vi "RIB Req - CJB Eathered Error - Normal Operation.vi"(0 "Limits File Path":path, 5 "Results File Path":path, 11 "error in":errorcluster) -> (4 "Results Data Array":string[][](array[string]), 15 "error out":errorcluster)   [LabVIEW 2024]
doc: "Template test"
uses:
  <vilib>/addons/_JKI Toolkits/State Machine/_JKI_lib_State_Machine.llb/Select State(s)_err__jki_lib_state_machine.vi
  <vilib>/addons/_JKI Toolkits/State Machine/_JKI_lib_State_Machine.llb/Select State(s)_bool__jki_lib_state_machine.vi
  <vilib>/addons/_JKI Toolkits/State Machine/_JKI_lib_State_Machine.llb/Periodic Trigger__ogtk__JKI-SM__jki_lib_state_machine.vi
  <userlib>/_OpenG.lib/file/file.llb/Strip Path Extension - String__ogtk.vi
  <vilib>/Utility/file.llb/Read Delimited Spreadsheet (string).vi
  <vilib>/Utility/file.llb/Write Delimited Spreadsheet (string).vi
  <userlib>/_OpenG.lib/file/file.llb/openg_file.lvlib
  <userlib>/_OpenG.lib/appcontrol/appcontrol.llb/openg_application_control.lvlib
  <userlib>/_OpenG.lib/time/time.llb/openg_time.lvlib
panel:
  out "State Value":string
  out "Wait for Start":bool
  out "Normal Operation":bool
  out "Timeout - Start State":dbl(slide) scale=0.0..15.0
  in  "eSTOP 1 State Error Test":string
  in  "eSTOP 1 State Test":string
  in  "Read Start":string
  in  "Read Set":string
  out "Timeout":dbl(slide) scale=0.0..60.0
  in  "eSTOP 1 Error Test":string
  in  "eSTOP 1 Test":string
  in  "connection ID":refnum<k16>
  in  "handle out":u64
  in  "Exit":bool
  # "Normal Operation"
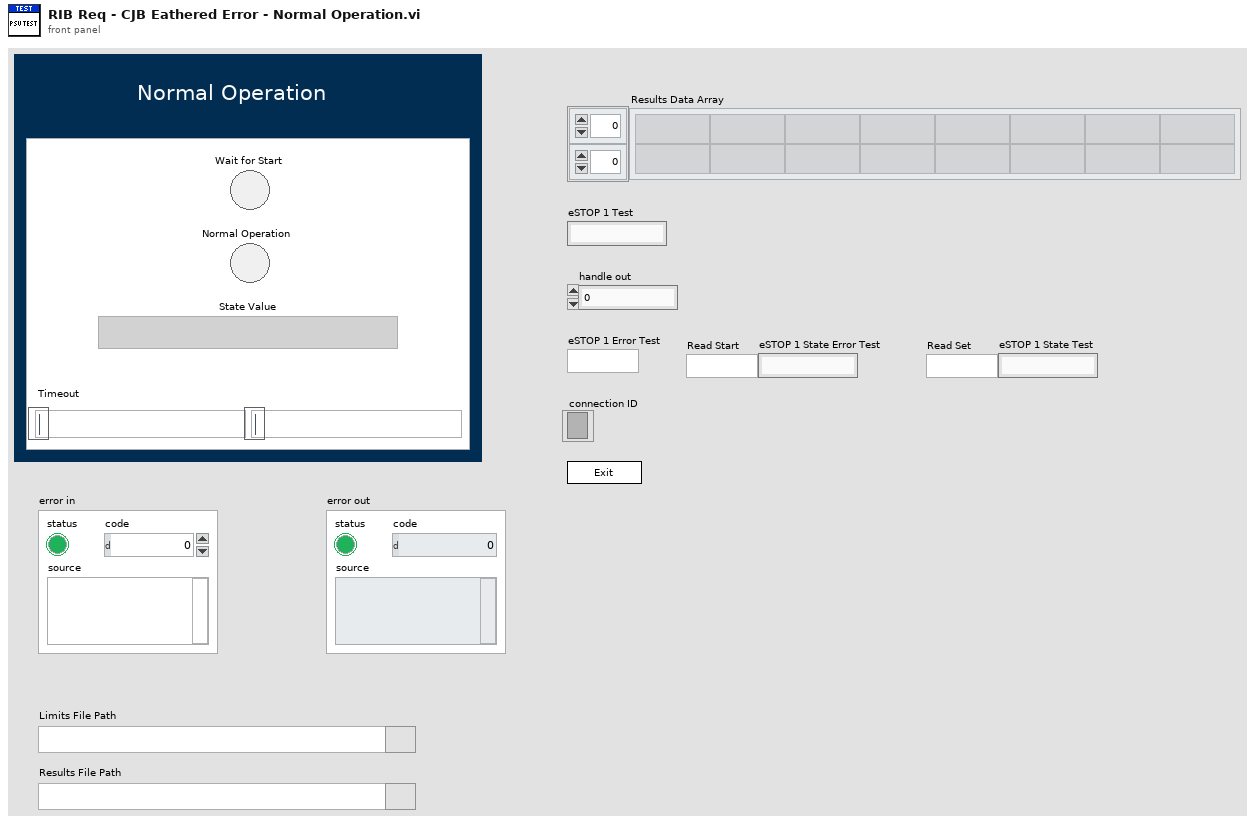
[diagram p1: front panel]
types:
  T1 = enum32{"Invalid", "Standard", "Closed", "Hidden", "Minimized", "Maximized"}
  T2 = enum32{"invalid app kind", "Development System", "Run Time System", "Student Edition", "Embedded LabVIEW", "Evaluation", "Custom"}
  T3 = typedef "FGV - Enum" = enum16{"Cleanup", "Get Data", "Simulator", "Open UDP", "Initialise DAQ", "Initialise I2C"}
  T4 = enum16{"Start Timer", "Get Time", "Pause", "Unpause"}
  T5 = cluster{"Core":cluster{"Current VI Reference":refnum<vi>, "Close Panel on Exit?":bool}, "Limits File Path":path, "Test Limits":string[][], "Results Data Array":string[][], "Results File Path":path, "Voltage":dbl, "connection ID":refnum<k16>, "handle out":u64, "eSTOP 1 Test":string, "eSTOP 1 Error Test":string, "Read Set":string, "Read Start ":string, "eSTOP 1 State Test":string, "eSTOP 1 State Error Test":string, "State Value":string}
  T6 = cluster{"Current VI Reference":refnum<vi>, "Close Panel on Exit?":bool}
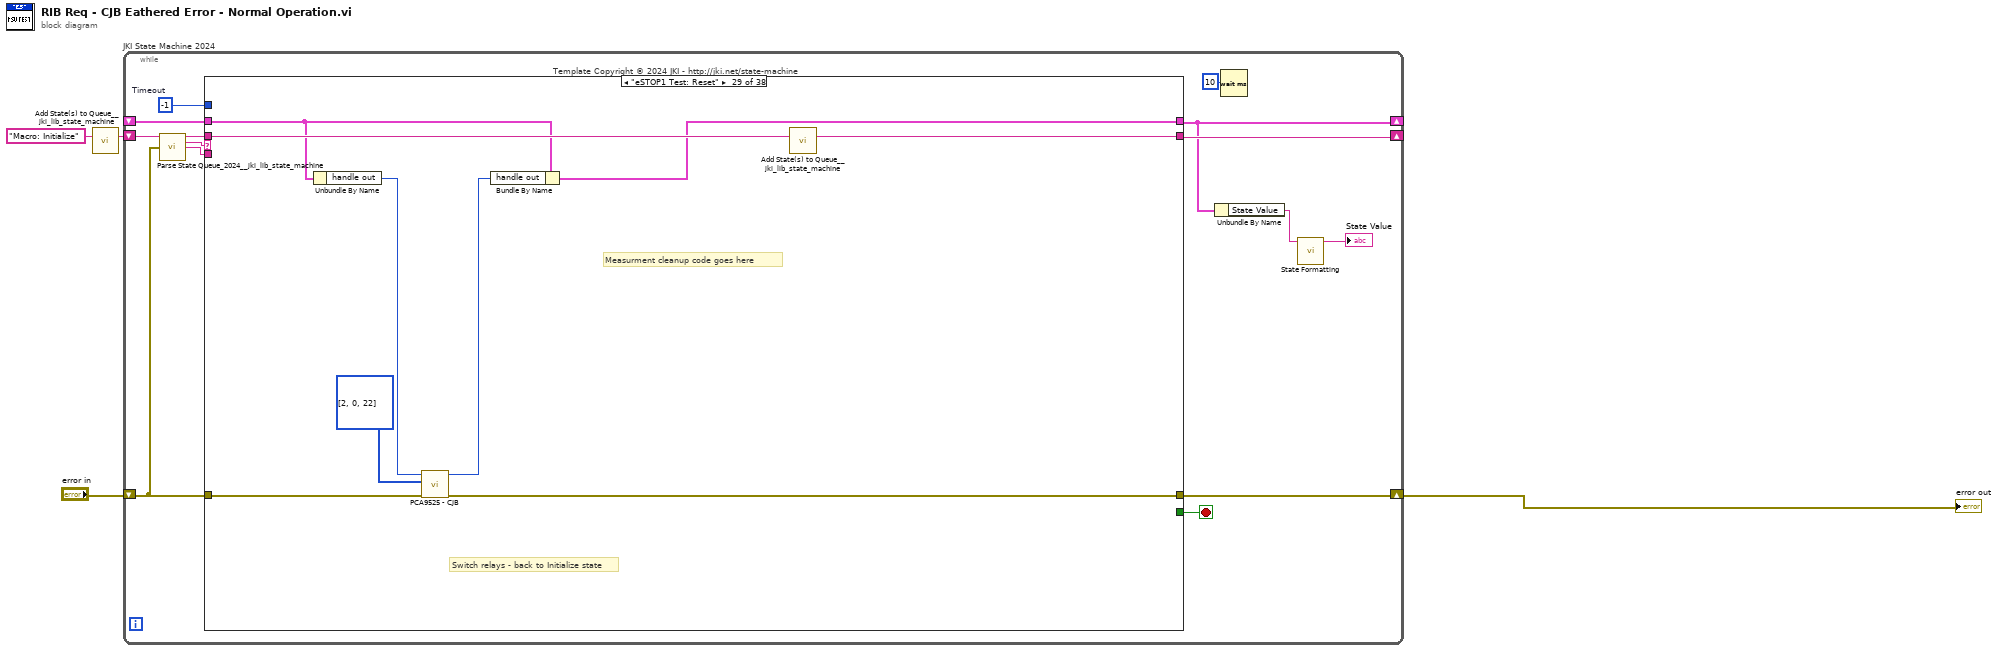
[diagram p0: block diagram]
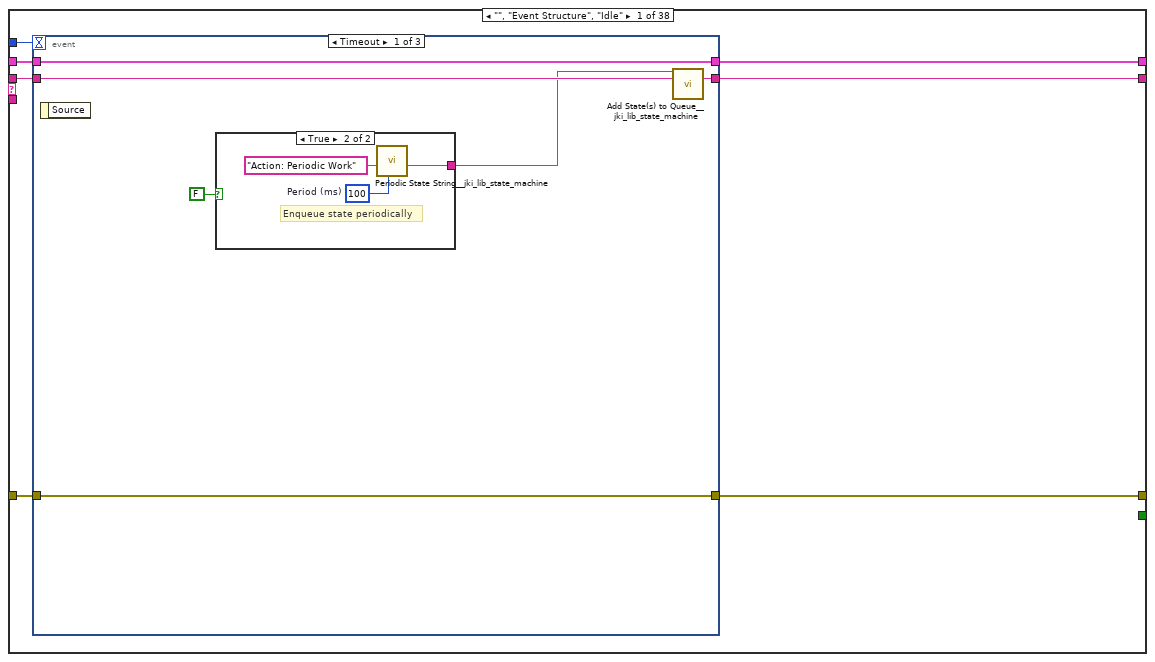
[diagram p2: hidden frame]
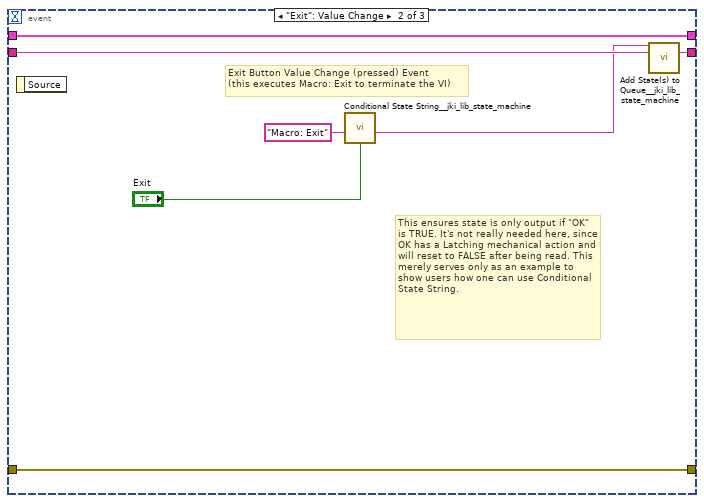
[diagram p4: hidden frame]
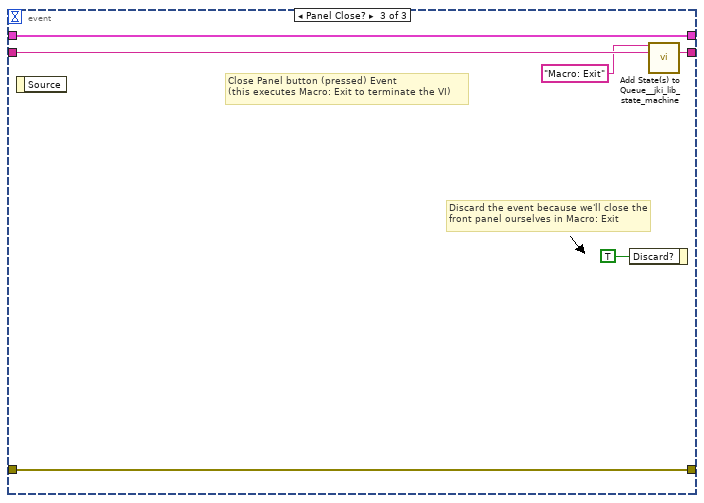
[diagram p5: hidden frame]
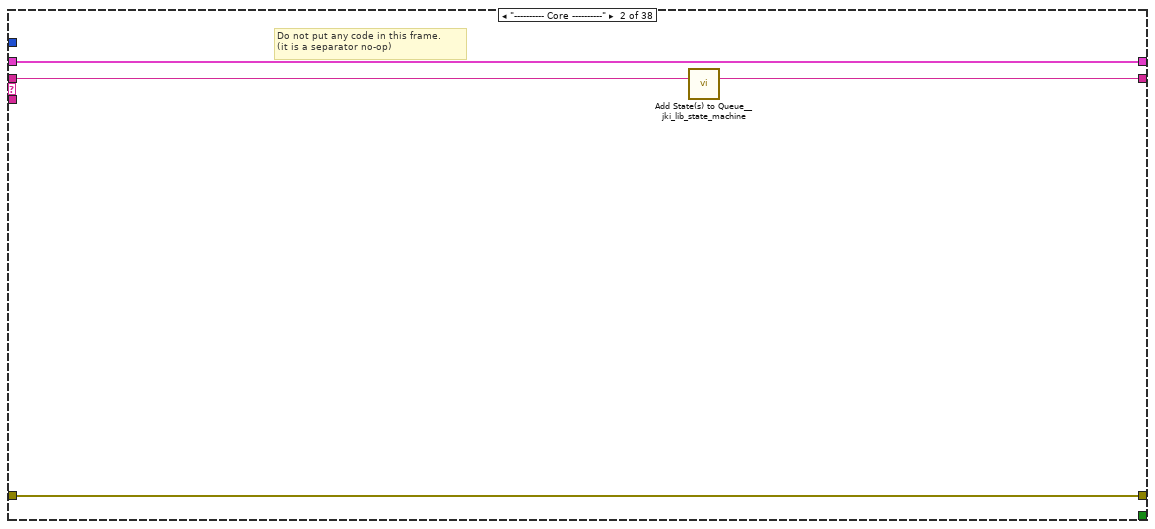
[diagram p6: hidden frame]
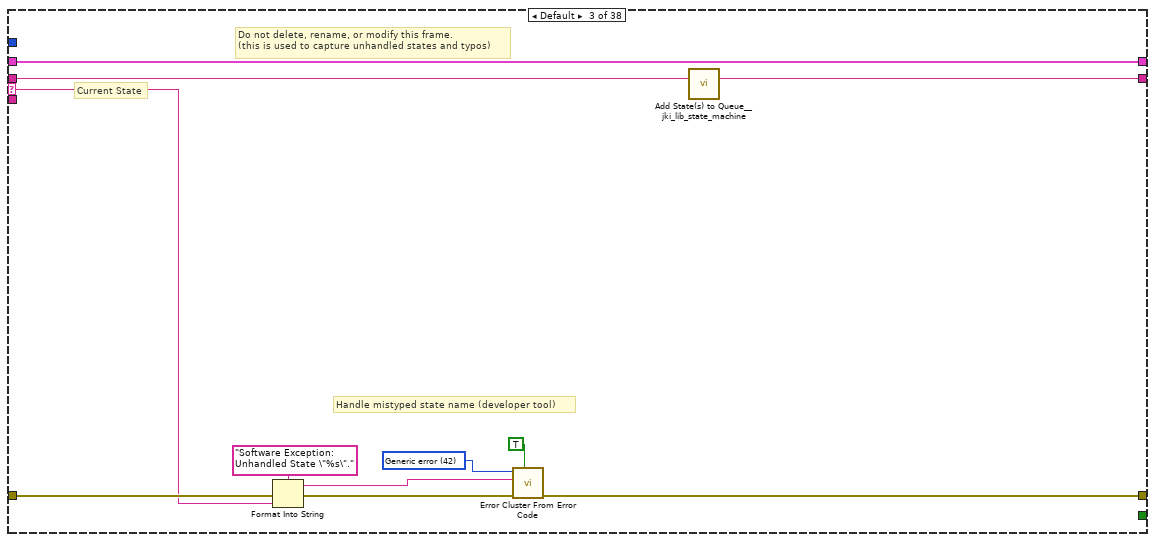
[diagram p7: hidden frame]
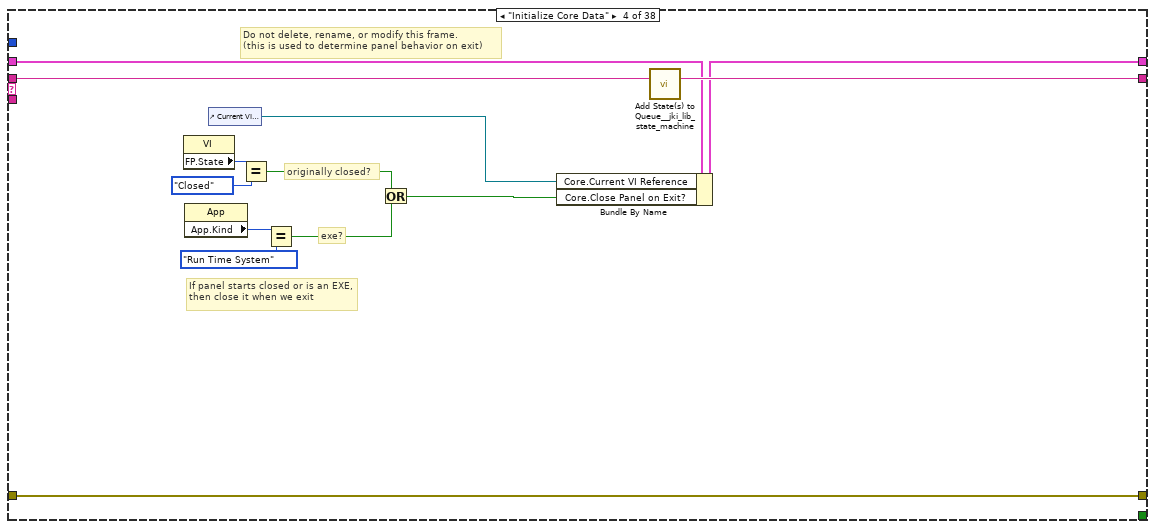
[diagram p8: hidden frame]
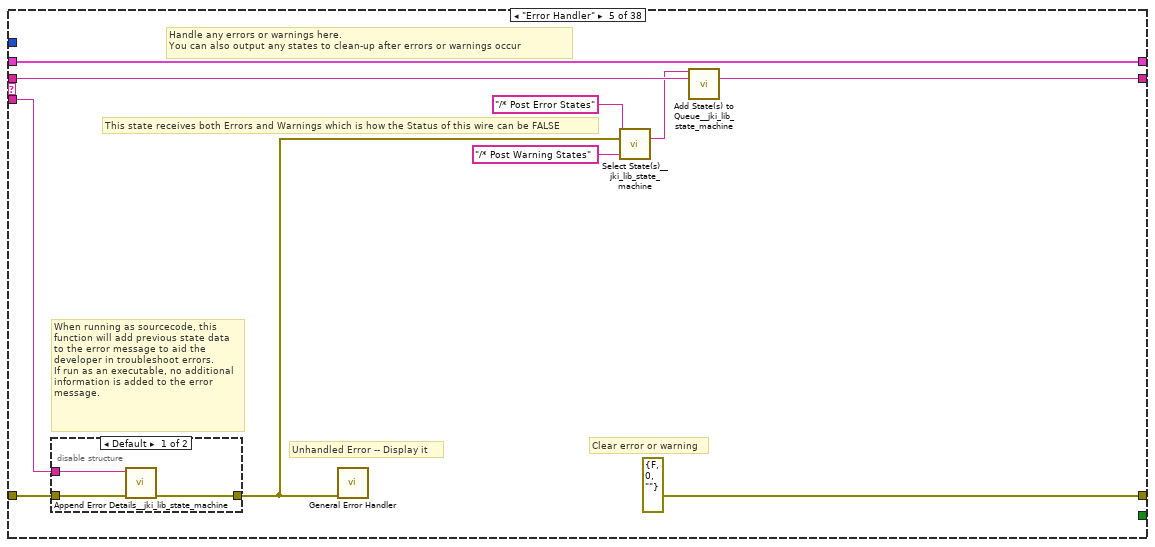
[diagram p9: hidden frame]
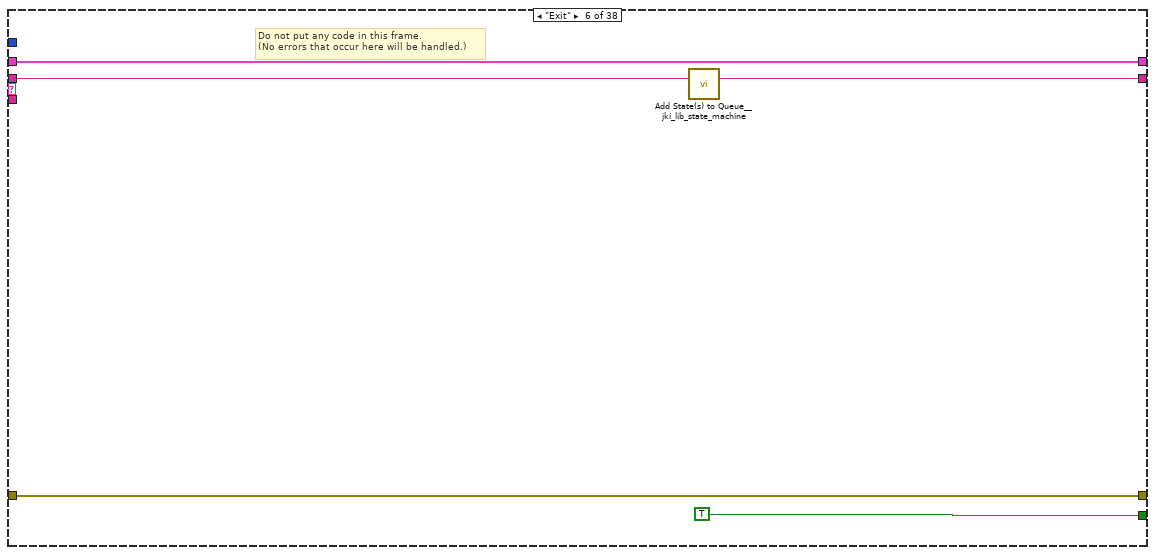
[diagram p11: hidden frame]
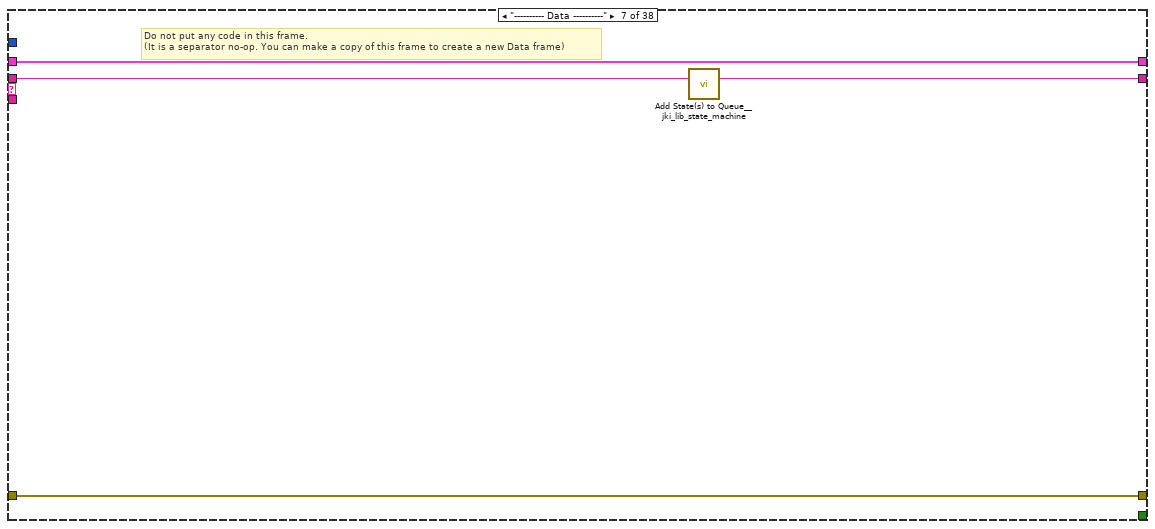
[diagram p12: hidden frame]
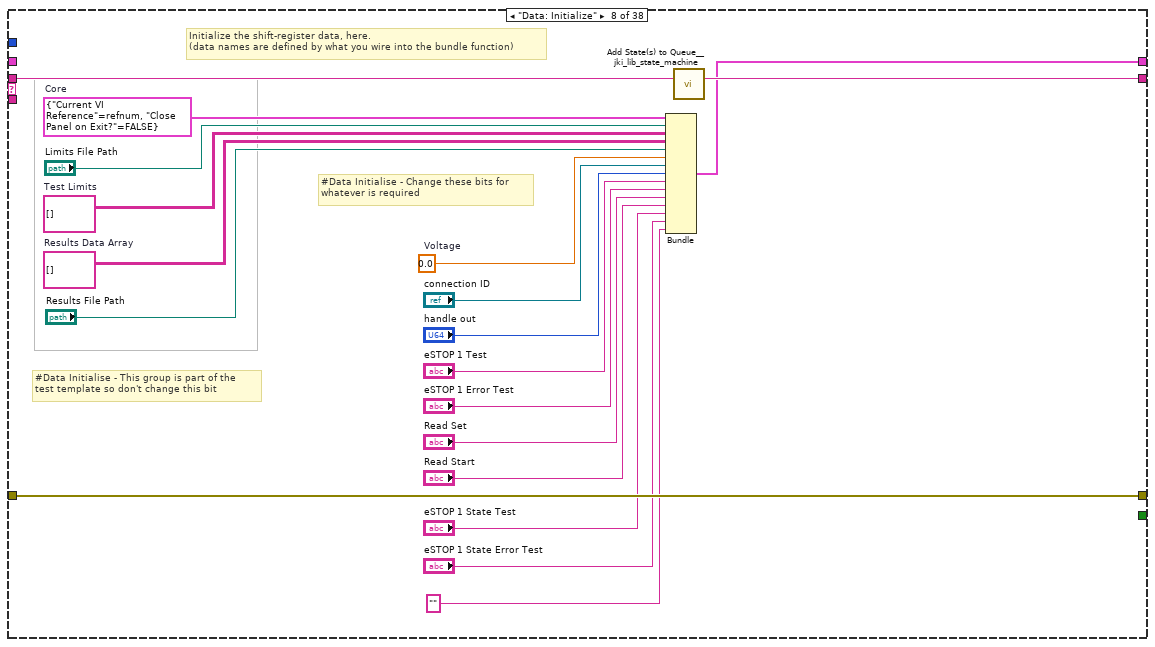
[diagram p13: hidden frame]
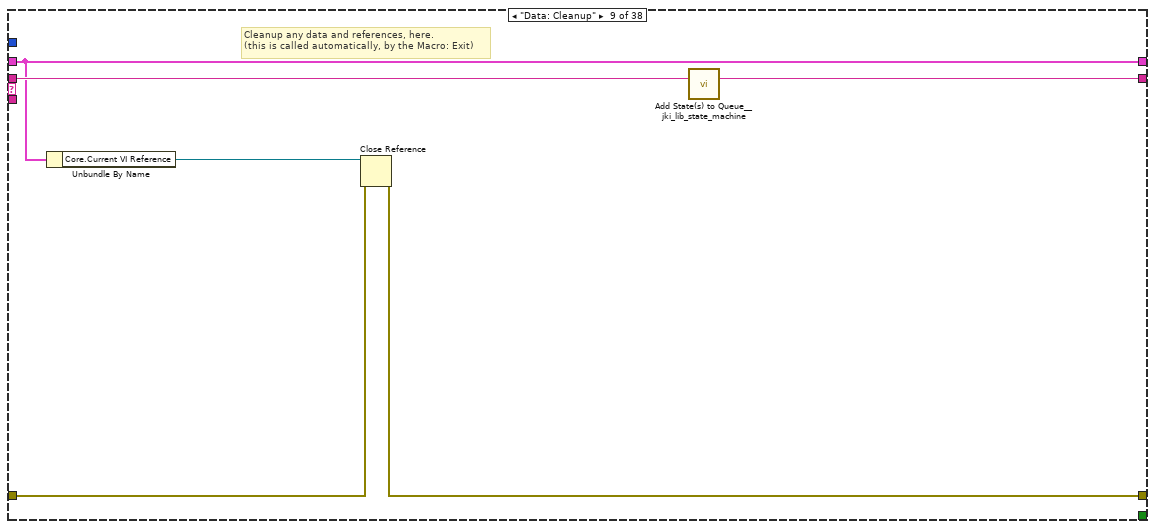
[diagram p14: hidden frame]
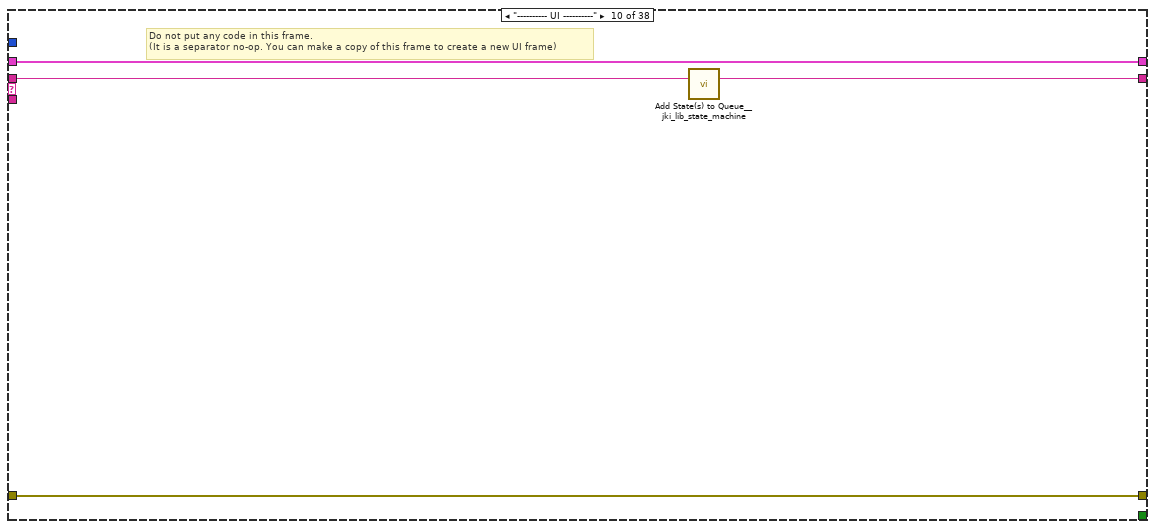
[diagram p15: hidden frame]
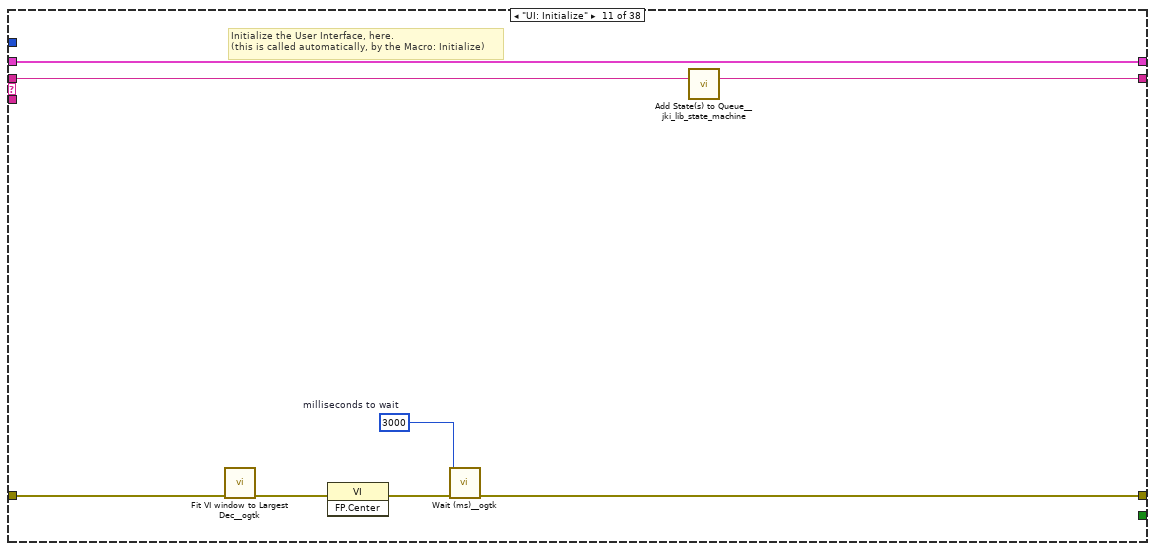
[diagram p16: hidden frame]
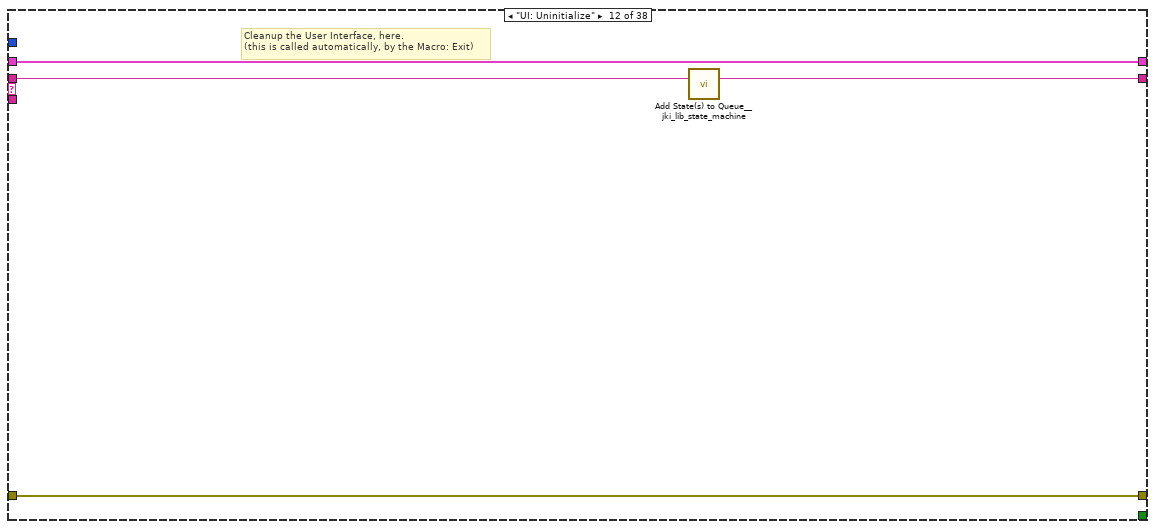
[diagram p17: hidden frame]
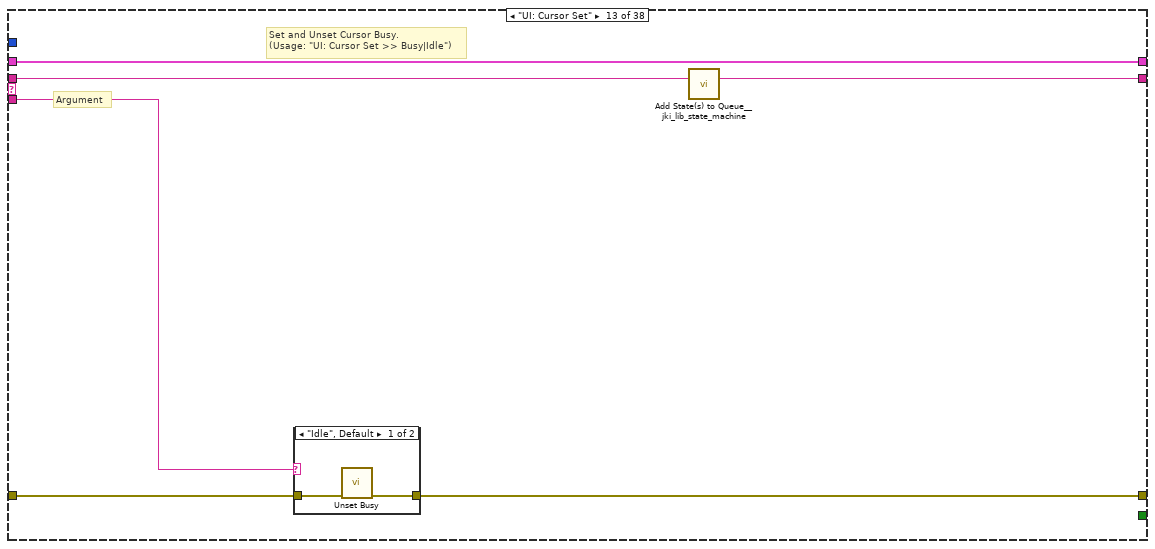
[diagram p18: hidden frame]
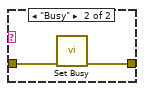
[diagram p19: hidden frame]
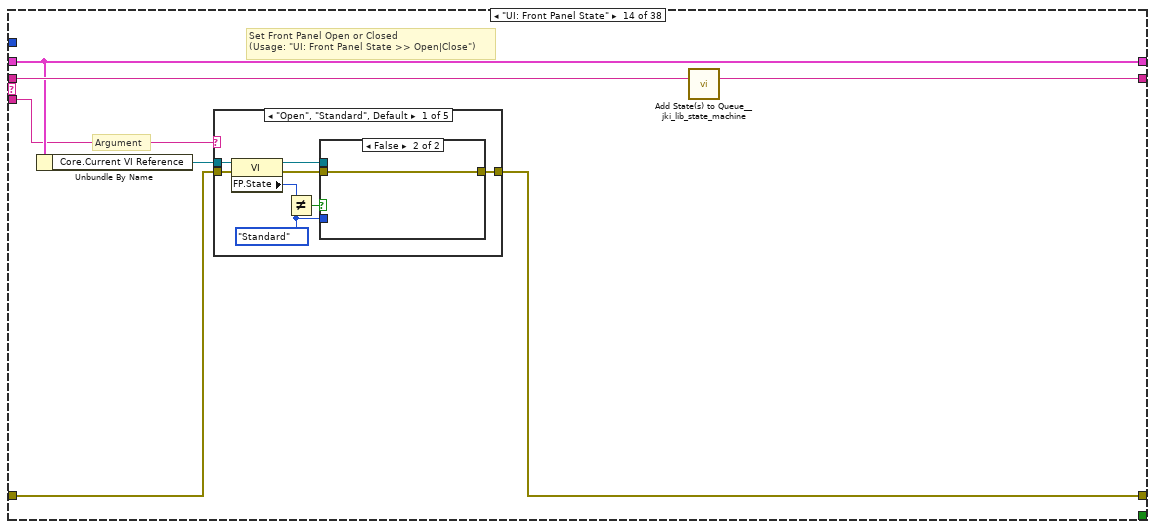
[diagram p20: hidden frame]
diagram:
  n1 = call <vilib>:"Add State(s) to Queue__jki_lib_state_machine.vi"("State(s) in (\"\")"="Macro: Initialize") -> ("States Out"=w4:string)  [unwired: 14 in]
  n2 = while "JKI State Machine 2024" {
    shift-right: [w5] -> _
    shift-left: _ -> [w11]
    shift-right: [w14] -> w1
    shift-left: "error in" -> [w9]
    shift-right: [w13] -> _
    shift-left: w4 -> [w15]
    stop <- w12 stop-if-true
    w10 = -1  # Timeout
    # "Template Copyright © 2024 JKI - http://jki.net/state-machine"
    n3 = call <vilib>:"Parse State Queue_2024__jki_lib_state_machine.vi"("State Queue"=w15, "Error In (no error)"=w9) -> ("Remaining States"=w17:string, "Current State"=w18:string, "Arguments"=w16:string)  [unwired: 11 in]
    n4 = case shown="\"eSTOP1 Test: Reset\"" w18 {
      selector: w18 -> [_ _ w52 _ _ _ _ _ _ _ _ _ _ _ _ _ _ _ _ _ _ _ _ _ _ _ _ _ _ _ _ _ _ _ _ _ _ _]
      tunnel: w17 -> [w25 w51 w56 w75 w85 w94 w98 w117 w123 w127 w135 w139 w145 w156 w225 w230 w235 w240 w245 w254 w258 w271 w288 w301 w305 w314 w318 w327 w336 w380 w399 w409 w432 w444 w463 w473 w496 w508]
      tunnel: w16 -> [_ _ _ _ w80 _ _ _ _ _ _ _ w140 w150 _ _ _ _ _ _ _ _ _ _ _ _ _ _ _ _ _ _ _ _ _ _ _ _]
      tunnel: w11 -> [w23 w48 w54 w68 w82 w92 w95 _ w118 w124 w133 w137 w143 w152 w222 w227 w232 w237 w242 w252 w255 w261 w280 w293 w302 w310 w315 w325 w334 w341 w396 w407 w429 w442 w460 w471 w493 w506]
      tunnel: [w22 w49 w58 w72 errorcluster {"status"=FALSE, "code"=0, "source"=""} ("error out") w91 w96 w114 w119 w125 w131 w136 w141 w153 w223 w228 w233 w238 w243 w249 w256 w267 w285 w298 w303 w312 w316 w322 w332 w338 w381 w400 w428 w436 w445 w464 w492 w500] -> w14
      tunnel: w9 -> [w19 w49 w57 w72 w81 w91 w96 w114 w120 w125 w132 w136 w142 w154 w223 w228 w233 w238 w243 w249 w256 w266 w284 w297 w303 w311 w316 w323 w331 w337 w395 w401 w428 w437 w459 w465 w492 w501]
      tunnel: [w24 w50 w55 w74 w84 w93 w97 w116 w122 w126 w134 w138 w144 w155 w224 w229 w234 w239 w244 w253 w257 w270 w287 w300 w304 w313 w317 w326 w335 w379 w398 w408 w431 w443 w462 w472 w495 w507] -> w13
      tunnel: [_ _ _ _ _ TRUE _ _ _ _ _ _ _ _ _ _ _ _ _ _ _ _ _ _ _ _ _ _ _ _ _ _ _ _ _ _ _ _] -> w12
      tunnel: [w21 w48 w54 w73 w82 w92 w95 w115 w118 w124 w133 w137 w143 w152 w222 w227 w232 w237 w242 w252 w255 w260 w279 w292 w302 w310 w315 w324 w333 w340 w397 w407 w430 w442 w461 w471 w494 w506] -> w5
      tunnel: w10 -> [w20 _ _ _ _ _ _ _ _ _ _ _ _ _ _ _ _ _ _ _ _ _ _ _ _ _ _ _ _ _ _ _ _ _ _ _ _ _]
      frame "", "Event Structure", "Idle" {
        n5 = event shown="[0] Timeout" {
          selector: _ -> [_ _ _]
          dyn-events: _ -> [_ _ _]
          timeout: w20 -> [_ _ _]
          tunnel: w25 -> [w31 w41 w47]
          tunnel: [w30 w40 w46] -> w24
          tunnel: w23 -> [w28 w38 w44]
          tunnel: [w29 w39 w45] -> w22
          tunnel: w19 -> [w29 w39 w45]
          tunnel: [w28 w38 w44] -> w21
          event Timeout {
            n6 = event-data() -> ()  [unwired: 1 in, 1 out]
            n7 = case shown="True" FALSE {
              tunnel: [_ w34] -> w27
              frame False {
              }
              frame True {
                w32 = u32 100  # Period (ms)
                # "Enqueue state periodically"
                n8 = call <vilib>:"Periodic State String__jki_lib_state_machine.vi"("Period (ms)"=w32, "State"="Action: Periodic Work") -> ("State Out"=w34:string)  [unwired: 9 in]
              }
            }
            n9 = call <vilib>:"Add State(s) to Queue__jki_lib_state_machine.vi"("State(s) in Front (\"\")"=w27, "State(s) in (\"\")"=w31) -> ("States Out"=w30:string)  [unwired: 13 in]
          }
          event "Exit": Value Change {
            # "This ensures state is only output if \"OK\" is TRUE. It's not really needed here, since OK has a Latching mechanical action and will reset to FALSE after being read. This merely serves only as an example to show users how one can use Conditional State String."
            # "Exit Button Value Change (pressed) Event\n(this executes Macro: Exit to terminate the VI)"
            n10 = event-data() -> ()  [unwired: 1 in, 1 out]
            n11 = call <vilib>:"Conditional State String__jki_lib_state_machine.vi"("Do State(s)?"="Exit", "State"="Macro: Exit") -> ("State Out"=w35:string)  [unwired: 7 in]
            n12 = call <vilib>:"Add State(s) to Queue__jki_lib_state_machine.vi"("State(s) in Front (\"\")"=w35, "State(s) in (\"\")"=w41) -> ("States Out"=w40:string)  [unwired: 13 in]
          }
          event Panel Close? {
            # "Discard the event because we'll close the front panel ourselves in Macro: Exit"
            # "Close Panel button (pressed) Event\n(this executes Macro: Exit to terminate the VI)"
            n13 = event-data() -> ()  [unwired: 1 in, 1 out]
            n14 = event-data("Discard?"=TRUE) -> ()  [unwired: 1 in, 1 out]
            n15 = call <vilib>:"Add State(s) to Queue__jki_lib_state_machine.vi"("State(s) in Front (\"\")"="Macro: Exit", "State(s) in (\"\")"=w47) -> ("States Out"=w46:string)  [unwired: 13 in]
          }
        }
      }
      frame "---------- Core ----------" {
        # "Do not put any code in this frame.\n(it is a separator no-op)"
        n16 = call <vilib>:"Add State(s) to Queue__jki_lib_state_machine.vi"("State(s) in (\"\")"=w51) -> ("States Out"=w50:string)  [unwired: 14 in]
      }
      frame Default {
        w61 = 42 items=["No error", "Argument error", "Memory is full", "Out of zone", "End of file", "File already open", "Generic file I/O error", "File not found", "File permission error", "Disk is full", "Duplicate path", "Too many files open", "System feature not enabled", "Resource file not found", "Cannot add resource", "Resource not found", "Image not found", "Image memory error", "Pen does not exist", "Config type invalid", "Config token not found", "Config parse error", "Config memory error", "Bad external code format", "Bad external code offset", "External code not present", "Null window", "Destroy window error", "Null menu", "Print aborted", "Bad print record", "Print driver error", "Windows error during printing", "Memory error during printing", "Print dialog error", "Generic print error", "Invalid device refnum", "Device not found", "Device parameter error", "Device unit error", "Cannot open device", "Device call aborted", "Generic error", "Cancelled by user", "Object ID too low", "Object ID too high", "Object not in heap", "Unknown heap", "Unknown object (invalid DefProc)", "Unknown object (DefProc not in table)", "Message out of range", "Invalid (null) method", "Unknown message", "Manager call not supported", "Bad address", "Network operation in progress", "Network operation timed out", "Connection is busy", "Network attribute not supported", "Network error", "Address in use", "System out of memory", "Connection aborted", "Connection refused", "Not connected", "Already connected", "Connection closed", "Initialization error (interapplication manager)", "Bad occurrence", "Wait on unbound occurrence handler", "Occurrence queue overflow", "Datalog type conflict", "Unused", "Unrecognized type (interapplication manager)", "Memory corrupt", "Failed to make temporary DLL", "Old CIN version", "Drag socket not found", "Failed to load drop-object", "Failed to register OLE object", "Failed to release OLE object", "Format specifier type mismatch", "Unknown format specifier", "Too few format specifiers", "Too many format specifiers", "Scan failed", "Newer CIN version", "Error converting to variant", "Runtime menu error", "Password tampered", "Variant attribute not found", "Incompatible variant data type", "Event data is not available", "Event Store is not present", "Occurrence is not found", "Event Queue is not created", "Event info is not available", "Refnum passed is NULL", "Error retrieving Class GUID", "Error retrieving CoClass GUID", "Error retrieving TypeLib GUID.", "Bad built application magic bytes.", "Specific driver is different from the specific driver associated with the Logical Name.", "There is no session opened to the class driver.", "Max Error", "MAX - Error with config objects", "MAX - Error loading configuration", "MAX - Group not supported"]
        # "Current State"
        # "Do not delete, rename, or modify this frame.\n(this is used to capture unhandled states and typos)"
        # "Handle mistyped state name (developer tool)"
        n17 = Format Into String(format string="Software Exception: Unhandled State \"%s\"." ("message"), error in=w57, w52) -> (resulting string=w60:string, error out=w59:errorcluster)  [unwired: 1 in]
        n18 = call <vilib>:"Error Cluster From Error Code.vi"("show call chain? (False)"=TRUE, "error in (no error)"=w59, "error message (\"\")"=w60, "error code (0)"=w61) -> ("error out"=w58:errorcluster)  [unwired: 5 in]
        n19 = call <vilib>:"Add State(s) to Queue__jki_lib_state_machine.vi"("State(s) in (\"\")"=w56) -> ("States Out"=w55:string)  [unwired: 14 in]
      }
      frame "Initialize Core Data" {
        # "Do not delete, rename, or modify this frame.\n(this is used to determine panel behavior on exit)"
        # "originally closed?"
        # "exe?"
        # "If panel starts closed or is an EXE, then close it when we exit"
        n20 = property class="VI"() -> ("FP.State"=w65:T1)  [unwired: 2 in, 2 out]
        n21 = property class="App"() -> ("App.Kind"=w71:T2)  [unwired: 2 in, 2 out]
        n22 = control-ref of="Current VI Reference"() -> (w66:refnum<vi>)
        n23 = Equal?(x=w65, y=T1."Closed" ("Front Panel Window:State")) -> (x = y?=w63:bool)
        n24 = Equal?(x=w71, y=T2."Run Time System" ("Application:Kind")) -> (x = y?=w69:bool)
        n25 = Or(x=w63, y=w69) -> (x .or. y?=w67:bool)
        n26 = Bundle By Name(cluster=w68, "Core.Current VI Reference"=w66, "Core.Close Panel on Exit?"=w67) -> (w73:T5)
        n27 = call <vilib>:"Add State(s) to Queue__jki_lib_state_machine.vi"("State(s) in (\"\")"=w75) -> ("States Out"=w74:string)  [unwired: 14 in]
      }
      frame "Error Handler" {
        # "When running as sourcecode, this function will add previous state data to the error message to aid the developer in troubleshoot errors.\nIf run as an executable, no additional information is added to the error message."
        # "This state receives both Errors and Warnings which is how the Status of this wire can be FALSE"
        # "Unhandled Error -- Display it"
        # "Handle any errors or warnings here.\nYou can also output any states to clean-up after errors or warnings occur"
        # "Clear error or warning"
        n28 = disable-structure shown="Default" {
          disable-tunnel: w81 -> [w88 w89]
          disable-tunnel: w80 -> [w87 _]
          disable-tunnel: [w86 w89] -> w79
          frame condition #0 (active) {
            n29 = call <vilib>:"Append Error Details__jki_lib_state_machine.vi"("error in (no error)"=w88, "Previous State and Argument(s)"=w87) -> ("error out"=w86:errorcluster)  [unwired: 9 in]
          }
          frame condition #1 {
          }
        }
        n30 = call <vilib>:"General Error Handler.vi"("error in (no error)"=w79) -> ()  [unwired: 10 in, 5 out]
        n31 = call-poly <vilib>:"Select State(s)__jki_lib_state_machine.vi"("State(s) if True (\"\")"="/* Post Error States", "Select"=w79, "State(s) if False (\"\")"="/* Post Warning States") -> ("States Out"=w77:string)  [unwired: 12 in]
        n32 = call <vilib>:"Add State(s) to Queue__jki_lib_state_machine.vi"("State(s) in Front (\"\")"=w77, "State(s) in (\"\")"=w85) -> ("States Out"=w84:string)  [unwired: 13 in]
      }
      frame "Exit" {
        # "Do not put any code in this frame.\n(No errors that occur here will be handled.)"
        n33 = call <vilib>:"Add State(s) to Queue__jki_lib_state_machine.vi"("State(s) in (\"\")"=w94) -> ("States Out"=w93:string)  [unwired: 14 in]
      }
      frame "---------- Data ----------" {
        # "Do not put any code in this frame.\n(It is a separator no-op. You can make a copy of this frame to create a new Data frame)"
        n34 = call <vilib>:"Add State(s) to Queue__jki_lib_state_machine.vi"("State(s) in (\"\")"=w98) -> ("States Out"=w97:string)  [unwired: 14 in]
      }
      frame "Data: Initialize" {
        w108 = 0.0  # Voltage
        w110 = string[][] []  # Results Data Array
        w111 = string[][] []  # Test Limits
        w113 = T6 {"Current VI Reference"=refnum, "Close Panel on Exit?"=FALSE}  # Core
        # "#Data Initialise - Change these bits for\nwhatever is required"
        # "#Data Initialise - This group is part of the\ntest template so don't change this bit"
        # "Initialize the shift-register data, here.\n(data names are defined by what you wire into the bundle function)"
        n35 = Bundle("Core"=w113, "Limits File Path"="Limits File Path", "Test Limits"=w111, "Results Data Array"=w110, "Results File Path"="Results File Path", "Voltage"=w108, "connection ID"="connection ID", "handle out"="handle out", "eSTOP 1 Test"="eSTOP 1 Test", "eSTOP 1 Error Test"="eSTOP 1 Error Test", "Read Set"="Read Set", "Read Start"="Read Start", "eSTOP 1 State Test"="eSTOP 1 State Test", "eSTOP 1 State Error Test"="eSTOP 1 State Error Test", "State Value"="") -> (w115:T5)  [unwired: 1 in]
        n36 = call <vilib>:"Add State(s) to Queue__jki_lib_state_machine.vi"("State(s) in (\"\")"=w117) -> ("States Out"=w116:string)  [unwired: 14 in]
      }
      frame "Data: Cleanup" {
        # "Cleanup any data and references, here.\n(this is called automatically, by the Macro: Exit)"
        n37 = Unbundle By Name(w118) -> ("Core.Current VI Reference"=w121:refnum<vi>)
        n38 = Close Reference(reference=w121, error in (no error)=w120) -> (error out=w119:errorcluster)
        n39 = call <vilib>:"Add State(s) to Queue__jki_lib_state_machine.vi"("State(s) in (\"\")"=w123) -> ("States Out"=w122:string)  [unwired: 14 in]
      }
      frame "---------- UI ----------" {
        # "Do not put any code in this frame.\n(It is a separator no-op. You can make a copy of this frame to create a new UI frame)"
        n40 = call <vilib>:"Add State(s) to Queue__jki_lib_state_machine.vi"("State(s) in (\"\")"=w127) -> ("States Out"=w126:string)  [unwired: 14 in]
      }
      frame "UI: Initialize" {
        w130 = u32 3000  # milliseconds to wait
        # "Initialize the User Interface, here.\n(this is called automatically, by the Macro: Initialize)"
        n41 = call <userlib>:"Fit VI window to Largest Dec__ogtk.vi"("error in (no error)"=w132) -> ("error out"=w128:errorcluster)  [unwired: 5 in, 1 out]
        n42 = invoke class="VI" method="FP.Center"(error in=w128) -> (error out=w129:errorcluster)  [unwired: 2 in, 2 out]
        n43 = call <userlib>:"Wait (ms)__ogtk.vi"("error in (no error)"=w129, "milliseconds to wait"=w130) -> ("error out"=w131:errorcluster)  [unwired: 8 in, 1 out]
        n44 = call <vilib>:"Add State(s) to Queue__jki_lib_state_machine.vi"("State(s) in (\"\")"=w135) -> ("States Out"=w134:string)  [unwired: 14 in]
      }
      frame "UI: Uninitialize" {
        # "Cleanup the User Interface, here.\n(this is called automatically, by the Macro: Exit)"
        n45 = call <vilib>:"Add State(s) to Queue__jki_lib_state_machine.vi"("State(s) in (\"\")"=w139) -> ("States Out"=w138:string)  [unwired: 14 in]
      }
      frame "UI: Cursor Set" {
        # "Argument"
        # "Set and Unset Cursor Busy.\n(Usage: \"UI: Cursor Set >> Busy|Idle\")"
        n46 = case shown="\"Idle\", Default" w140 {
          tunnel: w142 -> [w147 w149]
          tunnel: [w146 w148] -> w141
          frame "Idle", Default {
            n47 = call <vilib>:"Unset Busy.vi"("error in (no error)"=w147) -> ("error out"=w146:errorcluster)  [unwired: 10 in]
          }
          frame "Busy" {
            n48 = call <vilib>:"Set Busy.vi"("error in (no error)"=w149) -> ("error out"=w148:errorcluster)  [unwired: 9 in, 1 out]
          }
        }
        n49 = call <vilib>:"Add State(s) to Queue__jki_lib_state_machine.vi"("State(s) in (\"\")"=w145) -> ("States Out"=w144:string)  [unwired: 14 in]
      }
      frame "UI: Front Panel State" {
        # "Argument"
        # "Set Front Panel Open or Closed\n(Usage: \"UI: Front Panel State >> Open|Close\")"
        n50 = Unbundle By Name(w152) -> ("Core.Current VI Reference"=w151:refnum<vi>)
        n51 = case shown="\"Open\", \"Standard\", Default" w150 {
          tunnel: w154 -> [w162 w177 w188 w201 w214]
          tunnel: [w164 w178 w190 w203 w216] -> w153
          tunnel: w151 -> [w163 w175 w189 w202 w215]
          frame "Open", "Standard", Default {
            w157 = T1."Standard" ("State")
            n52 = property class="VI"(reference=w163, error in=w162) -> (reference out=w160:refnum<vi>, error out=w161:errorcluster, "FP.State"=w159:T1)
            n53 = Not Equal?(x=w159, y=w157) -> (x != y?=w158:bool)
            n54 = case shown="False" w158 {
              tunnel: [w168 w170] -> w164
              tunnel: w161 -> [w167 w170]
              tunnel: w160 -> [w166 _]
              tunnel: w157 -> [w165 _]
              frame True {
                n55 = invoke class="VI" method="FP.Open"(reference=w166, error in=w167, "Activate"=TRUE, "State"=w165) -> (error out=w168:errorcluster)  [unwired: 1 in, 4 out]
              }
              frame False {
              }
            }
          }
          frame "Close", "Closed" {
            n56 = property class="VI"(reference=w175, error in=w177) -> (reference out=w174:refnum<vi>, error out=w176:errorcluster, "FP.State"=w172:T1)
            n57 = Not Equal?(x=w172, y=T1."Closed" ("Front Panel Window:State")) -> (x != y?=w171:bool)
            n58 = case shown="True" w171 {
              tunnel: [w179 w182] -> w178
              tunnel: w176 -> [w179 w181]
              tunnel: w174 -> [_ w180]
              frame False {
              }
              frame True {
                n59 = invoke class="VI" method="FP.Close"(reference=w180, error in=w181) -> (error out=w182:errorcluster)  [unwired: 1 in, 2 out]
              }
            }
          }
          frame "Hidden", "Hide" {
            w183 = T1."Hidden" ("State")
            n60 = property class="VI"(reference=w189, error in=w188) -> (reference out=w186:refnum<vi>, error out=w187:errorcluster, "FP.State"=w185:T1)
            n61 = Not Equal?(x=w185, y=w183) -> (x != y?=w184:bool)
            n62 = case shown="True" w184 {
              tunnel: [w194 w195] -> w190
              tunnel: w187 -> [w193 w195]
              tunnel: w186 -> [w192 _]
              tunnel: w183 -> [w191 _]
              frame True {
                n63 = invoke class="VI" method="FP.Open"(reference=w192, error in=w193, "State"=w191) -> (error out=w194:errorcluster)  [unwired: 2 in, 4 out]
              }
              frame False {
              }
            }
          }
          frame "Minimize", "Minimized" {
            w196 = T1."Minimized" ("State")
            n64 = property class="VI"(reference=w202, error in=w201) -> (reference out=w199:refnum<vi>, error out=w200:errorcluster, "FP.State"=w198:T1)
            n65 = Not Equal?(x=w198, y=w196) -> (x != y?=w197:bool)
            n66 = case shown="True" w197 {
              tunnel: [w207 w208] -> w203
              tunnel: w200 -> [w206 w208]
              tunnel: w199 -> [w205 _]
              tunnel: w196 -> [w204 _]
              frame True {
                n67 = invoke class="VI" method="FP.Open"(reference=w205, error in=w206, "State"=w204) -> (error out=w207:errorcluster)  [unwired: 2 in, 4 out]
              }
              frame False {
              }
            }
          }
          frame "Maximize", "Maximized" {
            w209 = T1."Maximized" ("State")
            n68 = property class="VI"(reference=w215, error in=w214) -> (reference out=w212:refnum<vi>, error out=w213:errorcluster, "FP.State"=w211:T1)
            n69 = Not Equal?(x=w211, y=w209) -> (x != y?=w210:bool)
            n70 = case shown="True" w210 {
              tunnel: [w220 w221] -> w216
              tunnel: w213 -> [w219 w221]
              tunnel: w212 -> [w218 _]
              tunnel: w209 -> [w217 _]
              frame True {
                n71 = invoke class="VI" method="FP.Open"(reference=w218, error in=w219, "State"=w217) -> (error out=w220:errorcluster)  [unwired: 2 in, 4 out]
              }
              frame False {
              }
            }
          }
        }
        n72 = call <vilib>:"Add State(s) to Queue__jki_lib_state_machine.vi"("State(s) in (\"\")"=w156) -> ("States Out"=w155:string)  [unwired: 14 in]
      }
      frame "---------- Macro ----------" {
        # "Do not put any code in this frame.\n(It is a separator no-op. You can make a copy of this frame to create a new Macro frame)"
        n73 = call <vilib>:"Add State(s) to Queue__jki_lib_state_machine.vi"("State(s) in (\"\")"=w225) -> ("States Out"=w224:string)  [unwired: 14 in]
      }
      frame "Macro: Initialize" {
        # "Initialization Macro\n(This is called once, when the VI starts)"
        n74 = call <vilib>:"Add State(s) to Queue__jki_lib_state_machine.vi"("State(s) in Front (\"\")"="Data: Initialize\nInitialize Core Data\nUI: Initialize\nUI: Front Panel State >> Open\neSTOP1 Test: Initialise\nMacro: Test", "State(s) in (\"\")"=w230) -> ("States Out"=w229:string)  [unwired: 13 in]
      }
      frame "Macro: Test" {
        # "#Test Macro - Add the sequence \nfor measurments and limits testing here"
        n75 = call <vilib>:"Add State(s) to Queue__jki_lib_state_machine.vi"("State(s) in Front (\"\")"="Limits Test: Read Limits File\neSTOP1 Test: Reset\neSTOP1 Test: Disable ROV A B TMS\neSTOP1 Test: Set Command\neSTOP1 Test: Start Timer (Set)\neSTOP1 Test: Set Read Command", "State(s) in (\"\")"=w235) -> ("States Out"=w234:string)  [unwired: 13 in]
      }
      frame "Macro: Test 2" {
        # "#Test Macro - Add the sequence \nfor measurments and limits testing here"
        n76 = call <vilib>:"Add State(s) to Queue__jki_lib_state_machine.vi"("State(s) in Front (\"\")"="eSTOP1 Test: Start Command\neSTOP1 Test: Start Timer (Start)\neSTOP1 Test: Start Read Command", "State(s) in (\"\")"=w240) -> ("States Out"=w239:string)  [unwired: 13 in]
      }
      frame "Macro: Limits" {
        # "Do not put any code in this frame.\n(It is a separator no-op. You can make a copy of this frame to create a new Macro frame)"
        n77 = call <vilib>:"Add State(s) to Queue__jki_lib_state_machine.vi"("State(s) in Front (\"\")"="Limits Test: Read Set\nLimits Test: Read Start\nResults Data: Write Results Data\nMacro: Exit", "State(s) in (\"\")"=w245) -> ("States Out"=w244:string)  [unwired: 13 in]
      }
      frame "Macro: Exit" {
        # "Exit Macro\n(This is called once, when the VI exits)"
        n78 = Unbundle By Name(w252) -> ("Core.Close Panel on Exit?"=w247:bool)
        n79 = call <vilib>:"Conditional State String__jki_lib_state_machine.vi"("Do State(s)?"=w247, "State"="UI: Front Panel State >> Close") -> ("State Out"=w246:string)  [unwired: 7 in]
        n80 = call <vilib>:"Add State(s) to Queue__jki_lib_state_machine.vi"("State(s) in (\"\")"=w246, "State(s) at Back (\"\")"="UI: Uninitialize\nData: Cleanup\nExit") -> ("States Out"=w250:string)  [unwired: 13 in]
        n81 = call <vilib>:"Add State(s) to Queue__jki_lib_state_machine.vi"("State(s) in Front (\"\")"=w250, "State(s) in (\"\")"=w254) -> ("States Out"=w253:string)  [unwired: 13 in]
      }
      frame "---------- Limits Test ----------" {
        # "Template Separator\n(You can make a copy of, or modify, this frame)"
        n82 = call <vilib>:"Add State(s) to Queue__jki_lib_state_machine.vi"("State(s) in (\"\")"=w258) -> ("States Out"=w257:string)  [unwired: 14 in]
      }
      frame "Limits Test: Read Limits File" {
        w264 = ","  # delimiter (\t)
        n83 = Unbundle By Name(w261) -> ("Limits File Path"=w265:path)
        n84 = Current VI's Path "Test Case Path"() -> (path=w269:path)
        n85 = call-poly <vilib>:"Read Delimited Spreadsheet.vi"("file path (dialog if empty)"=w265, "error in (no error)"=w266, "delimiter (\\t)"=w264) -> ("all rows"=w262:string[][], "error out"=w267:errorcluster)  [unwired: 7 in, 4 out]
        n86 = Strip Path(path=w269) -> (name=w268:string)  [unwired: 1 out]
        n87 = call-poly <userlib>:"Strip Path Extension__ogtk.vi"("path"=w268) -> ("root"=w263:string)  [unwired: 1 out]
        n88 = for {
          tunnel: w263 -> [w275]
          tunnel: w262 -> [w273] mode=indexing
          tunnel: [w273] -> w259 mode=indexing if=w272
          n89 = Index Array(array=w273) -> (element=w274:string)  [unwired: 1 in]
          n90 = Equal?(x=w275, y=w274) -> (x = y?=w272:bool)
        }
        n91 = Bundle By Name(cluster=w261, "Test Limits"=w259) -> (w260:T5)
        n92 = call <vilib>:"Add State(s) to Queue__jki_lib_state_machine.vi"("State(s) in (\"\")"=w271) -> ("States Out"=w270:string)  [unwired: 14 in]
      }
      frame "Limits Test: Read Set" {
        w281 = "Read Set Test"  # Sub Test Name
        # "Equal to F1?"
        # "#Limits Testing - Add the sub test name for\ntest included in limits file"
        n93 = Unbundle By Name(w280) -> ("Results Data Array"=w278:string[][])
        n94 = Unbundle By Name(w280) -> ("Test Limits"=w282:string[][], "Read Set"=w286:string)
        n95 = To Variant(anything=w286) -> (Variant=w283:variant)
        n96 = call "Process Results.vi"("error in (no error)"=w284, "Measurement"=w283, "Test Limits"=w282, "Sub Test Name"=w281) -> ("error out"=w285:errorcluster, "Results Data"=w277:string[])  [unwired: 6 in]
        n97 = Build Array (concatenate)(w278, w277) -> (w276:string[][])
        n98 = Bundle By Name(cluster=w280, "Results Data Array"=w276) -> (w279:T5)
        n99 = call <vilib>:"Add State(s) to Queue__jki_lib_state_machine.vi"("State(s) in (\"\")"=w288) -> ("States Out"=w287:string)  [unwired: 14 in]
      }
      frame "Limits Test: Read Start" {
        w294 = "Read Start Test"  # Sub Test Name
        # "Equal to F1?"
        # "#Limits Testing - Add the sub test name for\ntest included in limits file"
        n100 = Unbundle By Name(w293) -> ("Results Data Array"=w291:string[][])
        n101 = Unbundle By Name(w293) -> ("Test Limits"=w295:string[][], "Read Start"=w299:string)
        n102 = To Variant(anything=w299) -> (Variant=w296:variant)
        n103 = call "Process Results.vi"("error in (no error)"=w297, "Measurement"=w296, "Test Limits"=w295, "Sub Test Name"=w294) -> ("error out"=w298:errorcluster, "Results Data"=w290:string[])  [unwired: 6 in]
        n104 = Build Array (concatenate)(w291, w290) -> (w289:string[][])
        n105 = Bundle By Name(cluster=w293, "Results Data Array"=w289) -> (w292:T5)
        n106 = call <vilib>:"Add State(s) to Queue__jki_lib_state_machine.vi"("State(s) in (\"\")"=w301) -> ("States Out"=w300:string)  [unwired: 14 in]
      }
      frame "---------- Results Data ----------" {
        # "Template Separator\n(You can make a copy of, or modify, this frame)"
        n107 = call <vilib>:"Add State(s) to Queue__jki_lib_state_machine.vi"("State(s) in (\"\")"=w305) -> ("States Out"=w304:string)  [unwired: 14 in]
      }
      frame "Results Data: Write Results Data" {
        w307 = ","  # delimiter (\t)
        w308 = TRUE  # append to file? (new file:F)
        n108 = Unbundle By Name(w310) -> ("Results File Path"=w309:path, "Results Data Array"=w306:string[][])
        "Results Data Array" <- w306
        n109 = call-poly <vilib>:"Write Delimited Spreadsheet.vi"("file path (dialog if empty)"=w309, "2D data"=w306, "append to file? (new file:F)"=w308, "error in (no error)"=w311, "delimiter (\\t)"=w307) -> ("error out"=w312:errorcluster)  [unwired: 9 in, 1 out]
        n110 = call <vilib>:"Add State(s) to Queue__jki_lib_state_machine.vi"("State(s) in (\"\")"=w314) -> ("States Out"=w313:string)  [unwired: 14 in]
      }
      frame "---------- eSTOP1 Test ----------" {
        # "Template Separator\n(You can make a copy of, or modify, this frame)"
        n111 = call <vilib>:"Add State(s) to Queue__jki_lib_state_machine.vi"("State(s) in (\"\")"=w318) -> ("States Out"=w317:string)  [unwired: 14 in]
      }
      frame "eSTOP1 Test: Initialise" {
        # "Measurement initialisation code goes here"
        n112 = call "FGV - Initialise.vi"("Enum"=FGV_-_Enum."Get Data", "Error In"=w323) -> ("connection ID"=w320:refnum<k16>, "Handle Out"=w319:u64, "Error Out"=w322:errorcluster)  [unwired: 13 in, 2 out]
        n113 = Bundle By Name(cluster=w325, "connection ID"=w320, "handle out"=w319) -> (w324:T5)
        n114 = call <vilib>:"Add State(s) to Queue__jki_lib_state_machine.vi"("State(s) in (\"\")"=w327) -> ("States Out"=w326:string)  [unwired: 14 in]
      }
      frame "eSTOP1 Test: Reset" {
        # "Switch relays - back to Initialize state"
        # "Measurment cleanup code goes here"
        n115 = Unbundle By Name(w334) -> ("handle out"=w329:u64)
        n116 = call "PCA9525 - CJB.vi"("error in (no error)"=w331, "buffer"=u8[] [2, 0, 22], "handle"=w329) -> ("error out"=w332:errorcluster, "handle out"=w328:u64)  [unwired: 7 in]
        n117 = Bundle By Name(cluster=w334, "handle out"=w328) -> (w333:T5)
        n118 = call <vilib>:"Add State(s) to Queue__jki_lib_state_machine.vi"("State(s) in (\"\")"=w336) -> ("States Out"=w335:string)  [unwired: 14 in]
      }
      frame "eSTOP1 Test: Disable ROV A B TMS" {
        w365 = u16 54321 ("port or service name")
        # "This is already tested and will speed up the test"
        # "Data"
        # "Length"
        # "ID"
        # "Target"
        # "Type"
        # "Pkt ID"
        # "Data"
        # "Length"
        # "ID"
        # "Target"
        # "Type"
        # "Pkt ID"
        # "Data"
        # "Length"
        # "ID"
        # "Target"
        # "Type"
        # "Pkt ID"
        # "Send disable ROV A B TMS command to RIB Box"
        # "Template Separator\n(You can make a copy of, or modify, this frame)"
        n119 = Unbundle By Name(w341) -> ("connection ID"=w339:refnum<k16>)
        n120 = Build Array(u8 91 ("element"), u8 1 ("element"), u8 9 ("element"), u8 105 ("element"), u8 1 ("element"), u8 0 ("element")) -> (w375:u8[])
        n121 = Byte Array To String(unsigned byte array=w375) -> (string=w372:string)
        n122 = String To IP(1:"192.168.0.20" ("name")) -> (0:w378:u32)
        n123 = UDP Write(address=w378, port or service name=w365, connection ID=w339, data in=w372, 8:w337, 9:1000 ("timeout ms (25000)")) -> (error out=w342:errorcluster, 3:w345:refnum<k16>)
        n124 = Build Array(u8 91 ("element"), u8 1 ("element"), u8 9 ("element"), u8 106 ("element"), u8 1 ("element"), u8 0 ("element")) -> (w376:u8[])
        n125 = Byte Array To String(unsigned byte array=w376) -> (string=w373:string)
        n126 = UDP Write(address=w378, port or service name=w365, connection ID=w345, data in=w373, 8:w342, 9:1000 ("timeout ms (25000)")) -> (error out=w348:errorcluster, 3:w346:refnum<k16>)
        n127 = Build Array(u8 91 ("element"), u8 1 ("element"), u8 9 ("element"), u8 107 ("element"), u8 1 ("element"), u8 0 ("element")) -> (w377:u8[])
        n128 = Byte Array To String(unsigned byte array=w377) -> (string=w374:string)
        n129 = UDP Write(address=w378, port or service name=w365, connection ID=w346, data in=w374, 8:w348, 9:1000 ("timeout ms (25000)")) -> (error out=w344:errorcluster, 3:w347:refnum<k16>)
        n130 = Bundle By Name(cluster=w341, "connection ID"=w347) -> (w340:T5)
        n131 = call <userlib>:"Wait (ms)__ogtk.vi"("error in (no error)"=w344, "milliseconds to wait"=u32 1000) -> ("error out"=w338:errorcluster)  [unwired: 8 in, 1 out]
        n132 = call <vilib>:"Add State(s) to Queue__jki_lib_state_machine.vi"("State(s) in (\"\")"=w380) -> ("States Out"=w379:string)  [unwired: 14 in]
      }
      frame "eSTOP1 Test: Set Command" {
        # "Data"
        # "Length"
        # "ID"
        # "Target"
        # "Type"
        # "Pkt ID"
        # "Measurement initialisation code goes here"
        n133 = Unbundle By Name(w396) -> ("connection ID"=w394:refnum<k16>)
        n134 = Build Array(u8 91 ("element"), u8 1 ("element"), u8 9 ("element"), u8 108 ("element"), u8 0 ("element")) -> (w388:u8[])
        n135 = String To IP(1:"192.168.0.20" ("name")) -> (0:w392:u32)
        n136 = Byte Array To String(unsigned byte array=w388) -> (string=w382:string)
        n137 = UDP Write(address=w392, port or service name=u16 54321, connection ID=w394, data in=w382, 8:w395, 9:1000 ("timeout ms (25000)")) -> (error out=w381:errorcluster, 3:w393:refnum<k16>)
        n138 = Bundle By Name(cluster=w396, "connection ID"=w393) -> (w397:T5)
        n139 = call <vilib>:"Add State(s) to Queue__jki_lib_state_machine.vi"("State(s) in (\"\")"=w399) -> ("States Out"=w398:string)  [unwired: 14 in]
      }
      frame "eSTOP1 Test: Start Timer (Set)" {
        # "Template Separator\n(You can make a copy of, or modify, this frame)"
        n140 = call "Timer.vi"("error in (no error)"=w401, "Enum"=T4."Start Timer") -> ("error out"=w405:errorcluster)  [unwired: 6 in, 3 out]
        n141 = property on="Timeout" class="Slide (strict)"(error in=w405, "Value"=0.0 ("Horizontal Pointer Slide"), "Scale.Maximum"=20.0 ("Target Time"), "Scale.Minimum"=0.0 ("Scale.Range:Minimum")) -> (error out=w400:errorcluster)  [unwired: 1 in, 1 out]
        n142 = call <vilib>:"Add State(s) to Queue__jki_lib_state_machine.vi"("State(s) in (\"\")"=w409) -> ("States Out"=w408:string)  [unwired: 14 in]
      }
      frame "eSTOP1 Test: Set Read Command" {
        # "Read UDP if equal to F1 then test complete if false timer is check if elapsed"
        # "Measurement initialisation code goes here"
        n143 = Unbundle By Name(w429) -> ("connection ID"=w412:refnum<k16>)
        n144 = UDP Read(connection ID=w412, timeout ms (25000)=1) -> (data out=w415:string, error out=w418:errorcluster, 3:w413:refnum<k16>)  [unwired: 2 in, 2 out]
        n145 = String Subset(string=w415, offset (0)=17 ("offset (0) 2"), length (rest)=1 ("length (rest) 2")) -> (substring=w422:string)
        n146 = String To Byte Array(string=w422) -> (unsigned byte array=w427:u8[])
        n147 = Number To Hexadecimal String(2:w427) -> (0:w426:string[])  [unwired: 1 in]
        n148 = Index Array(array=w426, index=0) -> (element=w410:string)
        n149 = Equal?(x=w410, y="15") -> (x = y?=w414:bool)
        "Wait for Start" <- w414
        n150 = Bundle By Name(cluster=w429, "connection ID"=w413, "Read Set"=w410, "State Value"=w410) -> (w430:T5)
        n151 = call <vilib>:"Clear Errors.vi"("error in (no error)"=w418, "specific error code to clear (0: all)"=56) -> ()  [unwired: 4 in, 2 out]
        n152 = call-poly <vilib>:"Select State(s)__jki_lib_state_machine.vi"("State(s) if True (\"\")"="Macro: Test 2" ("State(s) if True (\"\")"), "Select"=w414, "State(s) if False (\"\")"="eSTOP1 Test: Elapsed Timer (Set)" ("State(s) if False (\"\")")) -> ("States Out"=w411:string)  [unwired: 12 in]
        n153 = call <vilib>:"Add State(s) to Queue__jki_lib_state_machine.vi"("State(s) in Front (\"\")"=w411, "State(s) in (\"\")"=w432) -> ("States Out"=w431:string)  [unwired: 13 in]
      }
      frame "eSTOP1 Test: Elapsed Timer (Set)" {
        # "check if timer elapsed if true end of test if false UDP is read again,"
        # "Template Separator\n(You can make a copy of, or modify, this frame)"
        n154 = call "Timer.vi"("error in (no error)"=w437, "Target Time"=20.0, "Enum"=T4."Get Time") -> ("error out"=w436:errorcluster, "Time Elapsed?"=w438:bool, "Elapsed Time"=→"Timeout":dbl)  [unwired: 5 in, 1 out]
        n155 = call-poly <vilib>:"Select State(s)__jki_lib_state_machine.vi"("State(s) if True (\"\")"="Macro: Test 2" ("State(s) if True (\"\")"), "Select"=w438, "State(s) if False (\"\")"="eSTOP1 Test: Set Read Command" ("State(s) if False (\"\")")) -> ("States Out"=w435:string)  [unwired: 12 in]
        n156 = call <vilib>:"Add State(s) to Queue__jki_lib_state_machine.vi"("State(s) in Front (\"\")"=w435, "State(s) in (\"\")"=w444) -> ("States Out"=w443:string)  [unwired: 13 in]
      }
      frame "eSTOP1 Test: Start Command" {
        # "Data"
        # "Length"
        # "ID"
        # "Target"
        # "Type"
        # "Pkt ID"
        # "Measurement initialisation code goes here"
        n157 = Unbundle By Name(w460) -> ("connection ID"=w458:refnum<k16>)
        n158 = Build Array(u8 91 ("element"), u8 1 ("element"), u8 9 ("element"), u8 110 ("element"), u8 0 ("element")) -> (w452:u8[])
        n159 = String To IP(1:"192.168.0.20" ("name")) -> (0:w456:u32)
        n160 = Byte Array To String(unsigned byte array=w452) -> (string=w446:string)
        n161 = UDP Write(address=w456, port or service name=u16 54321, connection ID=w458, data in=w446, 8:w459, 9:1000 ("timeout ms (25000)")) -> (error out=w445:errorcluster, 3:w457:refnum<k16>)
        n162 = Bundle By Name(cluster=w460, "connection ID"=w457) -> (w461:T5)
        n163 = call <vilib>:"Add State(s) to Queue__jki_lib_state_machine.vi"("State(s) in (\"\")"=w463) -> ("States Out"=w462:string)  [unwired: 14 in]
      }
      frame "eSTOP1 Test: Start Timer (Start)" {
        # "Template Separator\n(You can make a copy of, or modify, this frame)"
        n164 = call "Timer.vi"("error in (no error)"=w465, "Enum"=T4."Start Timer") -> ("error out"=w469:errorcluster)  [unwired: 6 in, 3 out]
        n165 = property on="Timeout - Start State" class="Slide (strict)"(error in=w469, "Value"=0.0 ("Horizontal Pointer Slide"), "Scale.Maximum"=15.0 ("Target Time"), "Scale.Minimum"=0.0 ("Scale.Range:Minimum")) -> (error out=w464:errorcluster)  [unwired: 1 in, 1 out]
        n166 = call <vilib>:"Add State(s) to Queue__jki_lib_state_machine.vi"("State(s) in (\"\")"=w473) -> ("States Out"=w472:string)  [unwired: 14 in]
      }
      frame "eSTOP1 Test: Start Read Command" {
        # "Read UDP if equal to F1 then test complete if false timer is check if elapsed"
        # "Measurement initialisation code goes here"
        n167 = Unbundle By Name(w493) -> ("connection ID"=w476:refnum<k16>)
        n168 = UDP Read(connection ID=w476, timeout ms (25000)=1) -> (data out=w479:string, error out=w482:errorcluster, 3:w477:refnum<k16>)  [unwired: 2 in, 2 out]
        n169 = String Subset(string=w479, offset (0)=17 ("offset (0) 2"), length (rest)=1 ("length (rest) 2")) -> (substring=w486:string)
        n170 = String To Byte Array(string=w486) -> (unsigned byte array=w491:u8[])
        n171 = Number To Hexadecimal String(2:w491) -> (0:w490:string[])  [unwired: 1 in]
        n172 = Index Array(array=w490, index=0) -> (element=w474:string)
        n173 = Equal?(x=w474, y="19") -> (x = y?=w478:bool)
        "Normal Operation" <- w478
        n174 = Bundle By Name(cluster=w493, "connection ID"=w477, "Read Start"=w474, "State Value"=w474) -> (w494:T5)
        n175 = call <vilib>:"Clear Errors.vi"("error in (no error)"=w482, "specific error code to clear (0: all)"=56) -> ()  [unwired: 4 in, 2 out]
        n176 = call-poly <vilib>:"Select State(s)__jki_lib_state_machine.vi"("State(s) if True (\"\")"="Macro: Limits" ("State(s) if True (\"\")"), "Select"=w478, "State(s) if False (\"\")"="eSTOP1 Test: Elapsed Timer (Start)" ("State(s) if False (\"\")")) -> ("States Out"=w475:string)  [unwired: 12 in]
        n177 = call <vilib>:"Add State(s) to Queue__jki_lib_state_machine.vi"("State(s) in Front (\"\")"=w475, "State(s) in (\"\")"=w496) -> ("States Out"=w495:string)  [unwired: 13 in]
      }
      frame "eSTOP1 Test: Elapsed Timer (Start)" {
        # "check if timer elapsed if true end of test if false UDP is read again,"
        # "Template Separator\n(You can make a copy of, or modify, this frame)"
        n178 = call "Timer.vi"("error in (no error)"=w501, "Target Time"=15.0, "Enum"=T4."Get Time") -> ("error out"=w500:errorcluster, "Time Elapsed?"=w502:bool, "Elapsed Time"=→"Timeout - Start State":dbl)  [unwired: 5 in, 1 out]
        n179 = call-poly <vilib>:"Select State(s)__jki_lib_state_machine.vi"("State(s) if True (\"\")"="Macro: Limits" ("State(s) if True (\"\")"), "Select"=w502, "State(s) if False (\"\")"="eSTOP1 Test: Start Read Command" ("State(s) if False (\"\")")) -> ("States Out"=w499:string)  [unwired: 12 in]
        n180 = call <vilib>:"Add State(s) to Queue__jki_lib_state_machine.vi"("State(s) in Front (\"\")"=w499, "State(s) in (\"\")"=w508) -> ("States Out"=w507:string)  [unwired: 13 in]
      }
    }
    n181 = Unbundle By Name(w5) -> ("State Value"=w6:string)
    n182 = Wait (ms)(milliseconds to wait=u32 10) -> ()  [unwired: 1 out]
    n183 = call "State Formatting.vi"("State Value 3"=w6) -> ("String"=→"State Value":string)  [unwired: 10 in]
  }
  "error out" <- w1
